vi "Line Tracking.vi"(0 "comm interface in":refnum<class "Pixy Com.lvclass">, 5 "features":enum16{"Main Features", "All Features"}(ring), 7 "feature map":u8=7 format="%.0x", 11 "error in":errorcluster) -> (4 "comm interface out":refnum<class "Pixy Com.lvclass">, 6 "vectors":T3[](array[typedef]), 8 "intersections":T2[](array[typedef]), 10 "barcodes":T1[](array[typedef]), 15 "error out":errorcluster)   [LabVIEW 2018, in "Pixy2.lvlib"]
uses:
  Pixy2.lvlib
  Interface/Pixy Com.lvclass
  Types/Vector.ctl
  Types/Intersection.ctl
  Types/Barcode.ctl
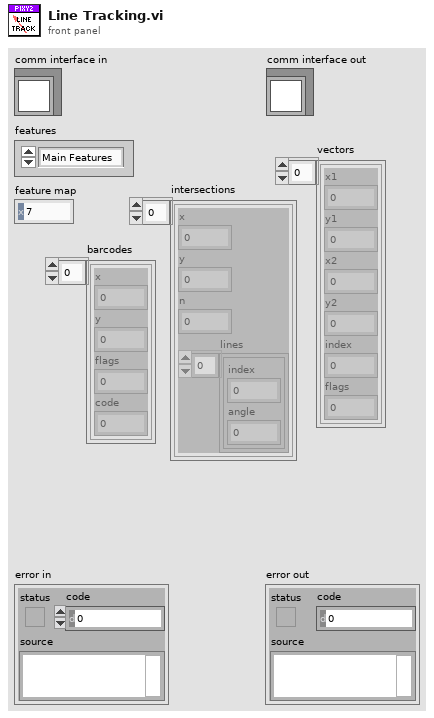
[diagram p1: front panel]
types:
  T1 = typedef "Pixy2.lvlib/Barcode.ctl" = cluster{"x":u8, "y":u8, "flags":u8, "code":u8}
  T2 = typedef "Pixy2.lvlib/Intersection.ctl" = cluster{"x":u8, "y":u8, "n":u8, "lines":cluster{"index":u8, "angle":i16}[]}
  T3 = typedef "Pixy2.lvlib/Vector.ctl" = cluster{"x1":u8, "y1":u8, "x2":u8, "y2":u8, "index":u8, "flags":u8}
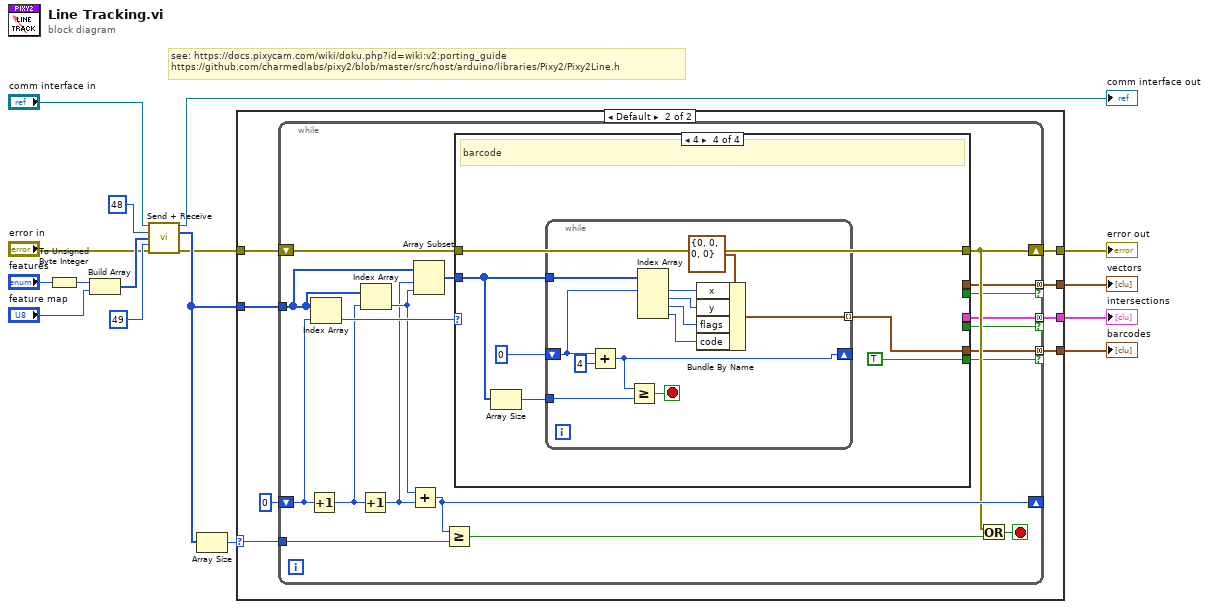
[diagram p0: block diagram]
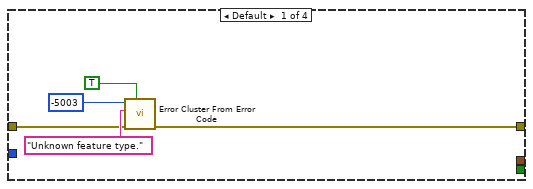
[diagram p3: hidden frame]
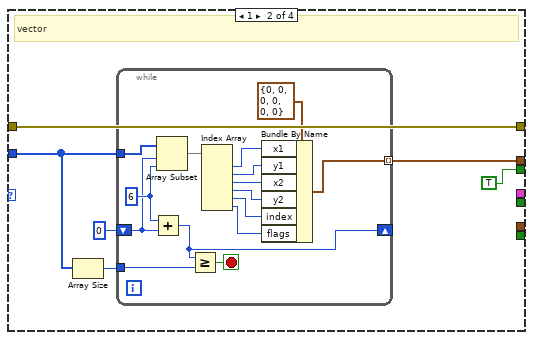
[diagram p4: hidden frame]
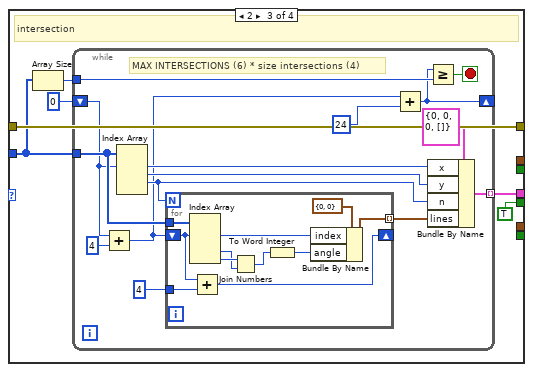
[diagram p5: hidden frame]
diagram:
  # "see: https://docs.pixycam.com/wiki/doku.php?id=wiki:v2:porting_guide\nhttps://github.com/charmedlabs/pixy2/blob/master/src/host/arduino/libraries/Pixy2/Pixy2Line.h"
  n1 = To Unsigned Byte Integer(number="features") -> (unsigned 8bit integer=w13:u8)
  n2 = Build Array(w13, "feature map") -> (w6:u8[])
  n3 = call "Send + Receive.vi"("comm interface in"="comm interface in", "type"=u8 48, "payload"=w6, "expected response"=u8 49 ("type"), "error in"="error in") -> ("comm interface out"=→"comm interface out":refnum<class "Pixy Com.lvclass">, "received"=w11:u8[], "error out"=w8:errorcluster)  [unwired: 8 in]
  n4 = Array Size(array=w11) -> (size(s)=w10:i32)
  n5 = case shown="Default" w10 {
    selector: w10 -> [_ w22]
    tunnel: [w17 w24] -> w12
    tunnel: w11 -> [_ w23]
    tunnel: [_ w21] -> w9
    tunnel: w8 -> [w17 w20]
    tunnel: [_ w19] -> w2
    tunnel: [_ w18] -> w1
    frame 0 {
    }
    frame Default {
      n6 = while {
        tunnel: w23 -> [w40]
        shift-right: [w35] -> _
        shift-left: 0 -> [w44]
        shift-right: [w34] -> w24
        shift-left: w20 -> [w42]
        tunnel: w22 -> [w36]
        tunnel: [w31] -> w21 mode=concatenating if=w30
        tunnel: [w29] -> w19 mode=concatenating if=w28
        tunnel: [w27] -> w18 mode=concatenating if=w26
        stop <- w32 stop-if-true
        n7 = Increment(x=w44) -> (x+1=w41:i32)
        n8 = Index Array(array=w40, index=w44) -> (element=w43:u8)
        n9 = Increment(x=w41) -> (x+1=w38:i32)
        n10 = Index Array(array=w40, index=w41) -> (element=w39:u8)
        n11 = Add(x=w39, y=w38) -> (x+y=w35:i32)
        n12 = Array Subset(array=w40, index=w38, length=w39) -> (w37:u8[])
        n13 = Greater Or Equal?(x=w35, y=w36) -> (x >= y?=w33:bool)
        n14 = case shown="4" w43 {
          tunnel: w42 -> [w46 w55 w76 w108]
          tunnel: w37 -> [_ w51 w72 w105]
          tunnel: [w45 w55 w76 w108] -> w34
          tunnel: [_ w54 _ _] -> w31
          tunnel: [_ TRUE _ _] -> w30
          tunnel: [_ _ w75 _] -> w29
          tunnel: [_ _ TRUE _] -> w28
          tunnel: [_ _ _ w107] -> w27
          tunnel: [_ _ _ TRUE] -> w26
          frame Default {
            n15 = call <vilib>:"Error Cluster From Error Code.vi"("show call chain? (False)"=TRUE, "error in (no error)"=w46, "error message (\"\")"="Unknown feature type." ("error message (\"\")"), "error code (0)"=-5003) -> ("error out"=w45:errorcluster)  [unwired: 5 in]
          }
          frame 1 {
            # "vector"
            n16 = Array Size(array=w51) -> (size(s)=w50:i32)
            n17 = while {
              tunnel: w51 -> [w62]
              tunnel: [w63] -> w54 mode=indexing
              shift-right: [w58] -> _
              shift-left: 0 -> [w56]
              tunnel: w50 -> [w59]
              stop <- w57 stop-if-true
              w60 = 6
              n18 = Add(x=w60, y=w56) -> (x+y=w58:i32)
              n19 = Array Subset(array=w62, index=w56, length=w60) -> (w61:u8[])
              n20 = Greater Or Equal?(x=w58, y=w59) -> (x >= y?=w57:bool)
              n21 = Index Array(array=w61) -> (element #1=w69:u8, element #2=w68:u8, element #3=w67:u8, element #4=w66:u8, element #5=w65:u8, element #6=w64:u8)  [unwired: 6 in]
              n22 = Bundle By Name(cluster=T3 {"x1"=0, "y1"=0, "x2"=0, "y2"=0, "index"=0, "flags"=0} ("vector"), "x1"=w69, "y1"=w68, "x2"=w67, "y2"=w66, "index"=w65, "flags"=w64) -> (w63:T3)
            }
          }
          frame 2 {
            # "intersection"
            n23 = Array Size(array=w72) -> (size(s)=w71:i32)
            n24 = while {
              tunnel: w72 -> [w88]
              tunnel: [w87] -> w75 mode=indexing
              shift-right: [w80] -> _
              shift-left: 0 -> [w83]
              tunnel: w71 -> [w82]
              stop <- w81 stop-if-true
              # "MAX INTERSECTIONS (6) * size intersections (4)"
              n25 = Add(x=w83, y=4) -> (x+y=w77:i32)
              n26 = Index Array(array=w88, index #1=w83) -> (element #1=w90:u8, element #2=w89:u8, element #3=w79:u8)  [unwired: 3 in, 1 out]
              n27 = for {
                N: w79 -> [_]
                tunnel: w88 -> [w102]
                shift-right: [w92] -> _
                shift-left: w77 -> [w94]
                tunnel: [w99] -> w86 mode=indexing
                tunnel: 4 -> [w93]
                n28 = Index Array(array=w102, index #1=w94) -> (element #1=w100:u8, element #3=w97:u8, element #4=w98:u8)  [unwired: 3 in, 1 out]
                n29 = Add(x=w94, y=w93) -> (x+y=w92:i32)
                n30 = Join Numbers(hi=w98, lo=w97) -> ((hi.lo)=w96:u16)
                n31 = To Word Integer(number=w96) -> (16bit integer=w95:i16)
                n32 = Bundle By Name(cluster=cluster{"index":u8, "angle":i16} {"index"=0, "angle"=0} ("vector"), "index"=w100, "angle"=w95) -> (w99:cluster{"index":u8, "angle":i16})
              }
              n33 = Add(x=w77, y=24 ("x")) -> (x+y=w80:i32)
              n34 = Greater Or Equal?(x=w80, y=w82) -> (x >= y?=w81:bool)
              n35 = Bundle By Name(cluster=T2 {"x"=0, "y"=0, "n"=0, "lines"=[]} ("intersection"), "x"=w90, "y"=w89, "n"=w79, "lines"=w86) -> (w87:T2)
            }
          }
          frame 4 {
            # "barcode"
            n36 = Array Size(array=w105) -> (size(s)=w103:i32)
            n37 = while {
              tunnel: w105 -> [w120]
              tunnel: [w114] -> w107 mode=indexing
              shift-right: [w110] -> _
              shift-left: 0 -> [w113]
              tunnel: w103 -> [w111]
              stop <- w109 stop-if-true
              n38 = Add(x=w113, y=4) -> (x+y=w110:i32)
              n39 = Greater Or Equal?(x=w110, y=w111) -> (x >= y?=w109:bool)
              n40 = Index Array(array=w120, index #1=w113) -> (element #1=w118:u8, element #2=w117:u8, element #3=w116:u8, element #4=w115:u8)  [unwired: 3 in]
              n41 = Bundle By Name(cluster=T1 {"x"=0, "y"=0, "flags"=0, "code"=0} ("barcode"), "x"=w118, "y"=w117, "flags"=w116, "code"=w115) -> (w114:T1)
            }
          }
        }
        n42 = Or(x=w34, y=w33) -> (x .or. y?=w32:bool)
      }
    }
  }
  "error out" <- w12
  "vectors" <- w9
  "intersections" <- w2
  "barcodes" <- w1
